vi "Sensor Interface Main.vi"(8 "error in (no error)":errorcluster) -> (0 "error out":errorcluster)   [LabVIEW 2020, in "Sensor Interface.lvlib"]
doc: "This is the Main VI for the Sensor Interface Module."
uses:
  Sensor Interface.lvlib
  Private Controls/FG Actions.ctl
  Private Controls/Module Data.ctl
  Private Controls/Message Cluster.ctl
  Private Controls/Message enum.ctl
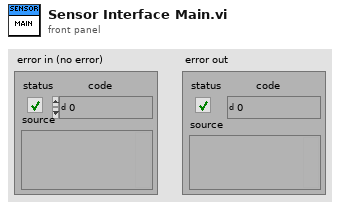
[diagram p1: front panel]
types:
  T1 = typedef "Sensor Interface.lvlib/Module Data.ctl" = cluster{"Data":variant}
  T2 = typedef "Sensor Interface.lvlib/FG Actions.ctl" = enum16{"Get", "Set", "Clear"}
  T3 = typedef "Sensor Interface.lvlib/Message Cluster.ctl" = cluster{"Message":T4, "Data":variant}
  T4 = typedef "Sensor Interface.lvlib/Message enum.ctl" = enum16{"Initialize", "State", "Error", "Exit"}
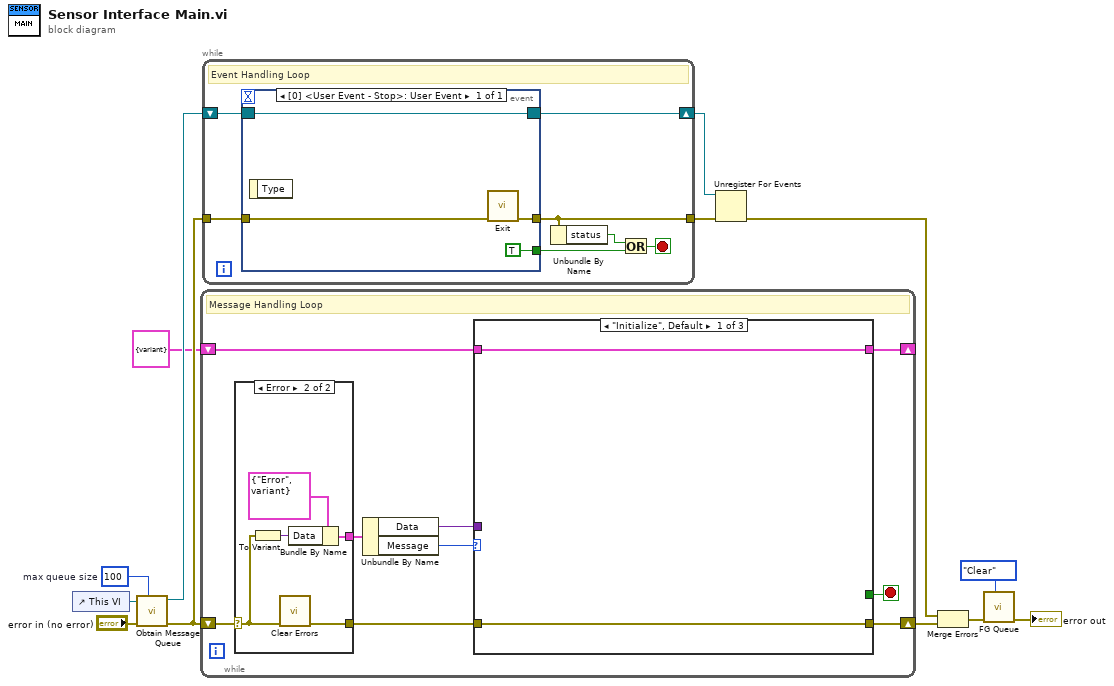
[diagram p0: block diagram]
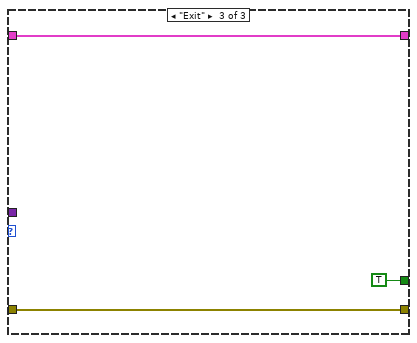
[diagram p3: hidden frame]
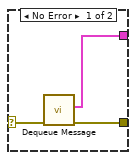
[diagram p4: hidden frame]
diagram:
  w7 = 100  # max queue size
  n1 = control-ref of="This VI"() -> (w8:refnum<vi>)
  n2 = call "Obtain Message Queue.vi"("max queue size (-1, unlimited)"=w7, "error in (no error)"="error in (no error)", "VI Reference"=w8) -> ("error out"=w3:errorcluster, "Event Registration Refnum"=w10:refnum<event-registration>)  [unwired: 7 in]
  n3 = while {
    shift-right: [w17] -> w13
    shift-left: w3 -> [w22]
    shift-right: [w14] -> _
    shift-left: T1 {"Data"=variant} ("Message Cluster") -> [w15]
    stop <- w16 stop-if-true
    # "Message Handling Loop"
    n4 = case shown="Error" w22 {
      selector: w22 -> [w30 w36]
      tunnel: [w31 w37] -> w18
      tunnel: [w32 w33] -> w21
      frame No Error {
        n5 = call "Dequeue Message.vi"("error in (no error)"=w30) -> ("error out"=w31:errorcluster, "Element"=w32:T3)  [unwired: 9 in]
      }
      frame Error {
        n6 = To Variant(anything=w36) -> (Variant=w34:variant)
        n7 = call <vilib>:"Clear Errors.vi"("error in (no error)"=w36) -> ("error out"=w37:errorcluster)  [unwired: 5 in, 1 out]
        n8 = Bundle By Name(cluster=T3 {"Message"=enum."Error", "Data"=variant} ("Message Cluster"), "Data"=w34) -> (w33:T3)
      }
    }
    n9 = Unbundle By Name(w21) -> ("Data"=w19:variant, "Message"=w20:T4)
    n10 = case shown="\"Initialize\", Default" w20 {
      tunnel: w19 -> [_ _ _]
      tunnel: w18 -> [w24 w26 w29]
      tunnel: [w24 w26 w29] -> w17
      tunnel: [_ _ TRUE] -> w16
      tunnel: w15 -> [w23 w25 w27]
      tunnel: [w23 w25 w27] -> w14
      frame "Initialize", Default {
      }
      frame "Error" {
      }
      frame "Exit" {
      }
    }
  }
  n11 = while {
    shift-right: [w43] -> w11
    shift-left: w10 -> [w44]
    tunnel: w3 -> [w41]
    tunnel: [w39] -> w2
    stop <- w40 stop-if-true
    # "Event Handling Loop"
    n12 = event shown="[0] <User Event - Stop>: User Event" {
      selector: w44 -> [w45]
      dyn-events: [w45] -> w43
      timeout: _ -> [_]
      tunnel: [TRUE ("Discard?")] -> w42
      tunnel: w41 -> [w47]
      tunnel: [w46] -> w39
      event User Event {
        n13 = event-data() -> ()  [unwired: 1 in, 1 out]
        n14 = call "Exit.vi"("error in (no error)"=w47) -> ("error out"=w46:errorcluster)  [unwired: 10 in]
      }
    }
    n15 = Unbundle By Name(w39) -> ("status"=w38:bool)
    n16 = Or(x=w38, y=w42) -> (x .or. y?=w40:bool)
  }
  n17 = Unregister For Events(event registration refnum=w11, error in=w2) -> (error out=w12:errorcluster)
  n18 = Merge Errors(w12, w13) -> (w5:errorcluster)
  n19 = call "FG Queue.vi"("FG Actions"=FG_Actions."Clear", "error in (no error)"=w5) -> ("error out"=→"error out":errorcluster)  [unwired: 8 in, 1 out]
